vi "Power_Factor.vi"() -> ()   [LabVIEW 2014]
panel:
  out "Irms":dbl
  in  "phase shift":dbl
  out "Power Factor":dbl
  out "Active Power P":dbl
  out "Reactive Power Q":dbl
  out "Vrms":dbl
  in  "current":dbl
  in  "Vin":dbl
  # "Ahmed Adel Hassan Elmashhor"
  # "Sec 1"
  # "Power Factor Calcs Drawn from a 3Phase Power Supply"
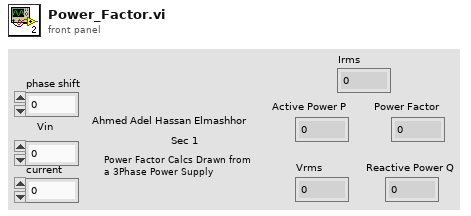
[diagram p1: front panel]
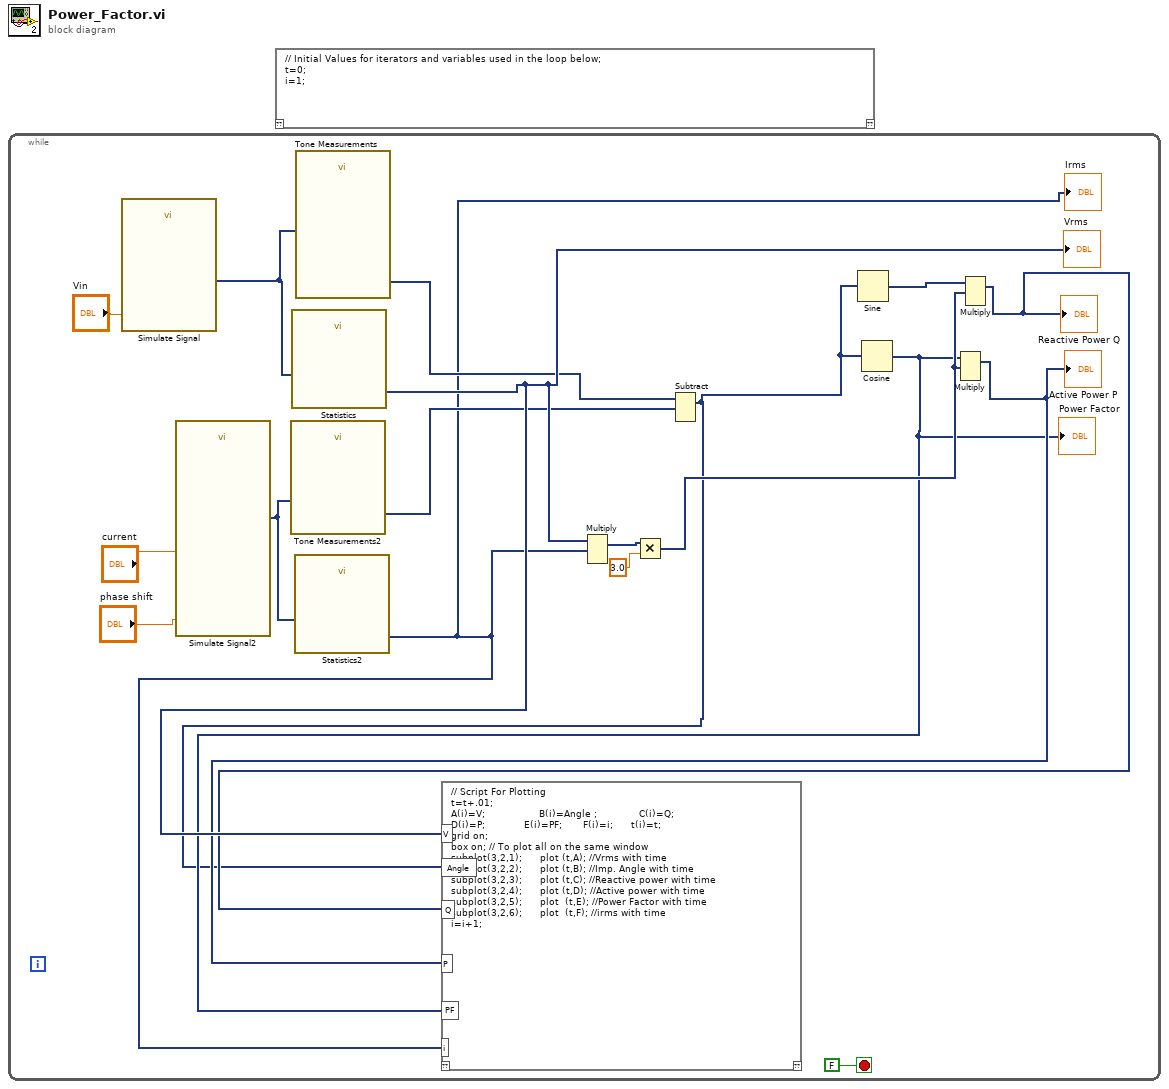
[diagram p0: block diagram]
diagram:
  n1 = while {
    stop <- FALSE stop-if-true
    n2 = call "Simulate Signal"("Amplitude"="Vin") -> ("Sine"=w15:dynamicdata)  [unwired: 13 in, 1 out]
    n3 = call "Simulate Signal2"("Amplitude"="current", "Phase"="phase shift") -> ("Sine"=w14:dynamicdata)  [unwired: 12 in, 1 out]
    n4 = call "Tone Measurements2"("Signals"=w14) -> ("Phase"=w3:dynamicdata)  [unwired: 9 in, 1 out]
    n5 = call "Statistics"("Signals"=w15) -> ("RMS"=w12:dynamicdata)  [unwired: 25 in, 1 out]
    "Vrms" <- w12
    n6 = call "Statistics2"("Signals"=w14) -> ("RMS"=w1:dynamicdata)  [unwired: 25 in, 1 out]
    "Irms" <- w1
    n7 = call "Tone Measurements"("Signals"=w15) -> ("Phase"=w2:dynamicdata)  [unwired: 9 in, 1 out]
    n8 = Multiply(1:w1, 2:w12) -> (0:w11:dynamicdata)  [unwired: 1 in, 1 out]
    n9 = Multiply(x=w11, y=3.0) -> (x*y=w9:dynamicdata)
    n10 = Subtract(1:w3, 2:w2) -> (0:w5:dynamicdata)  [unwired: 1 in, 1 out]
    n11 = Sine(x=w5) -> (sin(x)=w13:dynamicdata)
    n12 = Cosine(x=w5) -> (cos(x)=w6:dynamicdata)
    "Power Factor" <- w6
    n13 = Multiply(1:w9, 2:w6) -> (0:w7:dynamicdata)  [unwired: 1 in, 1 out]
    "Active Power P" <- w7
    n14 = Multiply(1:w9, 2:w13) -> (0:w8:dynamicdata)  [unwired: 1 in, 1 out]
    "Reactive Power Q" <- w8
    n15 = script code="// Script For Plotting\nt=t+.01;\nA(i)=V;                  B(i)=Angle ;              C(i)=Q;  \nD(i)=P;             E(i)=PF;       F(i)=i;      t(i)=t;\ngrid on;\nbox on; // To plot all on the same window\nsubplot(3,2,1);      plot (t,A); //Vrms with time\nsubplot(3,2,2);      plot (t,B); //Imp. Angle with time\nsubplot(3,2,3);      plot (t,C); //Reactive power with time\nsubplot(3,2,4);      plot (t,D); //Active power with time \nsubplot(3,2,5);      plot  (t,E); //Power Factor with time\nsubplot(3,2,6);      plot  (t,F); //irms with time\ni=i+1;"("V"=w12, "Angle"=w5, "Q"=w8, "P"=w7, "PF"=w6, "i"=w1) -> ()  [unwired: 1 in, 1 out]
  }
  n16 = script code="// Initial Values for iterators and variables used in the loop below;\nt=0;\ni=1;"() -> ()  [unwired: 1 in, 1 out]
